vi "AutoInit.vi"   [LabVIEW 2018]
uses:
  dsinstructions.vi
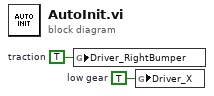
[diagram p0: block diagram]
diagram:
  w2 = TRUE  # low gear
  w1 = TRUE  # traction
  n1 = global write "dsinstructions.vi" "Driver_RightBumper"(w1) -> ()
  n2 = global write "dsinstructions.vi" "Driver_X"(w2) -> ()
